vi "Get Channel Range.vi"(8 "error in (no error)":errorcluster, 10 "Channel":T1, 11 "EPU452 in":refnum<class "EPU452.lvclass">) -> (0 "error out":errorcluster, 1 "Range":dbl, 2 "Response":string, 3 "EPU452 out":refnum<class "EPU452.lvclass">)   [LabVIEW 2018, in "EPU452.lvclass"]
uses:
  EPU452.lvclass
  Controls/Channels.ctl
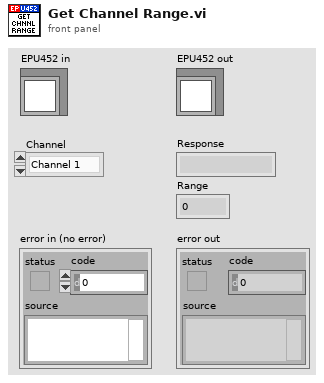
[diagram p1: front panel]
types:
  T1 = typedef "EPU452.lvclass/Channels.ctl" = enum16{"Channel 1", "Channel 2", "Channel 3", "Channel 4"}
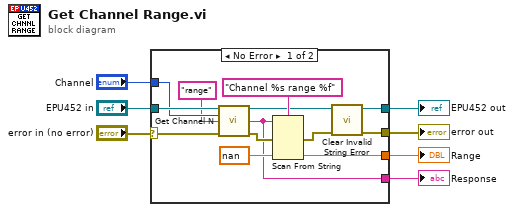
[diagram p0: block diagram]
diagram:
  n1 = case shown="No Error" "error in (no error)" {
    selector: "error in (no error)" -> [w8 w22]
    tunnel: [w9 w22] -> w6
    tunnel: [w10 w21] -> w4
    tunnel: "EPU452 in" -> [w20 w21]
    tunnel: "Channel" -> [w19 _]
    tunnel: [w13 _] -> w2
    tunnel: [w11 _] -> w1
    frame No Error {
      n2 = call "Get Channel N.vi"("EPU452 in"=w20, "Channel"=w19, "Function"="range", "error in (no error)"=w8) -> ("EPU452 out"=w14:refnum<class "EPU452.lvclass">, "Response"=w11:string, "error out"=w17:errorcluster)  [unwired: 9 in]
      n3 = Scan From String(format string="Channel %s range %f", input string=w11, error in=w17, default 2=nan ("default value 2")) -> (error out=w15:errorcluster, output 2=w13:dbl)  [unwired: 3 in, 2 out]
      n4 = call "Clear Invalid String Error.vi"("error in (no error)"=w15, "EPU452 in"=w14) -> ("error out"=w9:errorcluster, "EPU452 out"=w10:refnum<class "EPU452.lvclass">)  [unwired: 8 in]
    }
    frame Error {
    }
  }
  "error out" <- w6
  "EPU452 out" <- w4
  "Range" <- w2
  "Response" <- w1
